vi "Autonomous.vi"   [LabVIEW 2019]
doc: "This VI starts when autonomous period begins, and will automatically be terminated when it ends. You can carry out timed or sensor driven operations directly to I/O or to subsystems without needing to return to the caller."
uses:
  <vilib>/Rock Robotics/WPI/Utilities/WPI_GetSetVariantRefNum.vi
  <vilib>/Rock Robotics/Network Tables/NT Read String.vi
  <vilib>/Rock Robotics/Network Tables/NT Write String.vi
types:
  T1 = typedef "WPI_JoystickDevRef.ctl" = cluster{"Device":T2}
  T2 = typedef "WPI_JoystickDeviceEnum.ctl" = enum16{"USB 0", "USB 1", "USB 2", "USB 3", "USB 4", "USB 5"}
  T3 = typedef "Command Status Info.ctl" = cluster{"Name":string, "Status":T4, "notifier out":T5}
  T4 = typedef "Completion Status.ctl" = enum16{"Successful", "Aborted", "Incomplete"}
  T5 = typedef "Completion Notifier.ctl" = refnum<notifier>
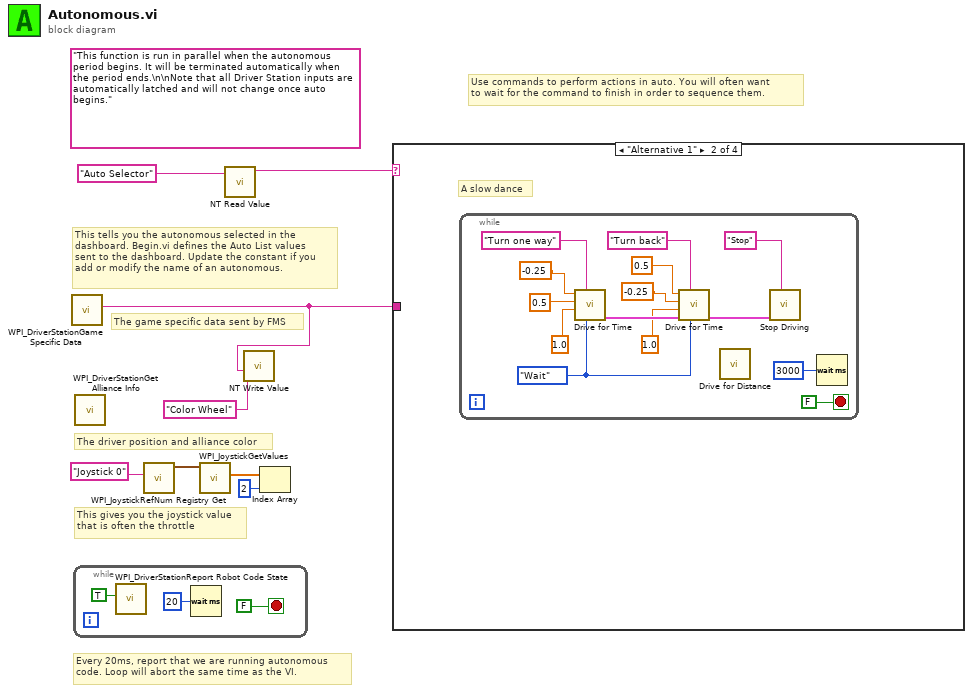
[diagram p0: block diagram]
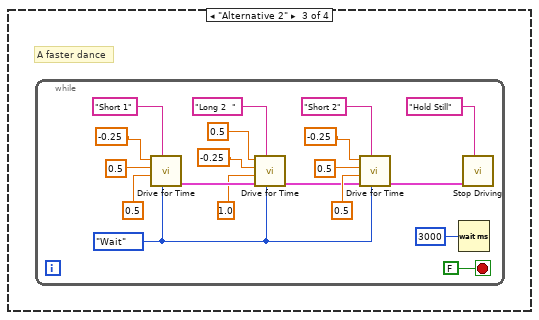
[diagram p3: hidden frame]
diagram:
  (unwired) "This function is run in parallel when the autonomous period begins. It will be terminated automatically when the period ends.\n\nNote that all Driver Station inputs are automatically latched and will not change once auto begins."
  # "The game specific data sent by FMS"
  # "This tells you the autonomous selected in the \ndashboard. Begin.vi defines the Auto List values\nsent to the dashboard. Update the constant if you\nadd or modify the name of an autonomous."
  # "Every 20ms, report that we are running autonomous\ncode. Loop will abort the same time as the VI."
  # "This gives you the joystick value\nthat is often the throttle"
  # "Use commands to perform actions in auto. You will often want\nto wait for the command to finish in order to sequence them."
  # "The driver position and alliance color"
  n1 = call <vilib>:"WPI_DriverStationGame Specific Data.vi"() -> ("Game Specific Data"=w2:string)  [unwired: 11 in]
  n2 = while {
    stop <- FALSE stop-if-true
    n3 = call <vilib>:"WPI_DriverStationReport Robot Code State.vi"("Autonomous"=TRUE) -> ()  [unwired: 10 in, 1 out]
    n4 = Wait (ms)(milliseconds to wait=u32 20) -> ()  [unwired: 1 out]
  }
  n5 = call <vilib>:"WPI_DriverStationGet Alliance Info.vi"() -> ()  [unwired: 12 out]
  n6 = call <vilib>:"WPI_JoystickRefNum Registry Get.vi"("refnum name"="Joystick 0") -> ("JoystickDevRef"=w7:T1)  [unwired: 1 in, 9 out]
  n7 = call <vilib>:"WPI_JoystickGetValues.vi"("JoystickDevRef"=w7) -> ("Axes"=w6:dbl[])  [unwired: 6 in, 4 out]
  n8 = call-poly <vilib>:"NT Read Value.vi"("Name"="Auto Selector") -> ("String"=w3:string)  [unwired: 9 in, 1 out]
  n9 = call-poly <vilib>:"NT Write Value.vi"("String"=w2, "Name"="Color Wheel") -> ()  [unwired: 9 in, 1 out]
  n10 = Index Array(array=w6, index=2) -> ()  [unwired: 1 out]
  n11 = case shown="\"Alternative 1\"" w3 {
    tunnel: w2 -> [_ _ _ _]
    frame Default {
      # "You can put your main auto here, or you can right-click on the case and make any\nother frame be the default case."
      # "This is the frame that will execute if no selection is made, or if it is not recognized"
    }
    frame "Alternative 1" {
      # "A slow dance"
      n12 = while {
        stop <- FALSE stop-if-true
        w16 = enum16{"Start", "Wait"}."Wait" ("Synchronication")
        n13 = call "Drive for Time.vi"("Synchronization"=w16, "Description"="Turn one way", "Seconds"=1.0 ("Delay (s)"), "Right Speed"=0.5 ("X axis value"), "Left Speed"=-0.25 ("X axis value")) -> ("Command Info Out"=w25:T3)  [unwired: 6 in]
        n14 = call "Drive for Time.vi"("Synchronization"=w16, "Description"="Turn back", "Command Info In"=w25, "Seconds"=1.0 ("Delay (s)"), "Right Speed"=-0.25 ("X axis value"), "Left Speed"=0.5 ("X axis value")) -> ("Command Info Out"=w15:T3)  [unwired: 5 in]
        n15 = call "Drive for Distance.vi"() -> ()  [unwired: 11 in, 1 out]
        n16 = call "Stop Driving.vi"("Description"="Stop", "Command Info In"=w15) -> ()  [unwired: 9 in, 1 out]
        n17 = Wait (ms)(milliseconds to wait=u32 3000 ("millisecond timer value")) -> ()  [unwired: 1 out]
      }
    }
    frame "Alternative 2" {
      # "A faster dance"
      n18 = while {
        stop <- FALSE stop-if-true
        w26 = enum16{"Start", "Wait"}."Wait" ("Synchronication")
        n19 = call "Drive for Time.vi"("Synchronization"=w26, "Description"="Short 1", "Seconds"=0.5 ("Delay (s)"), "Right Speed"=0.5 ("X axis value"), "Left Speed"=-0.25 ("X axis value")) -> ("Command Info Out"=w44:T3)  [unwired: 6 in]
        n20 = call "Drive for Time.vi"("Synchronization"=w26, "Description"="Long 2  ", "Command Info In"=w44, "Seconds"=1.0 ("Delay (s)"), "Right Speed"=-0.25 ("X axis value"), "Left Speed"=0.5 ("X axis value")) -> ("Command Info Out"=w28:T3)  [unwired: 5 in]
        n21 = call "Drive for Time.vi"("Synchronization"=w26, "Description"="Short 2", "Command Info In"=w28, "Seconds"=0.5 ("Delay (s)"), "Right Speed"=0.5 ("X axis value"), "Left Speed"=-0.25 ("X axis value")) -> ("Command Info Out"=w27:T3)  [unwired: 5 in]
        n22 = Wait (ms)(milliseconds to wait=u32 3000 ("millisecond timer value")) -> ()  [unwired: 1 out]
        n23 = call "Stop Driving.vi"("Description"="Hold Still", "Command Info In"=w27) -> ()  [unwired: 9 in, 1 out]
      }
    }
    frame "Your Turn" {
    }
  }
